vi "Renishaw-XL80_SetAutoCompensationMode.vi"(8 "error in (no error)":errorcluster, 10 "AutoCompensationMode":i32(ring) items=["AUTO_COMPENSATION_OFF"=0, "AUTO_COMPENSATION_AIR"=1, "AUTO_COMPENSATION_FULL"=3], 11 "Renishaw-XL80 in":refnum<class "Renishaw-XL80.lvclass">) -> (0 "error out":errorcluster, 3 "Renishaw-XL80 out":refnum<class "Renishaw-XL80.lvclass">)   [LabVIEW 2024, in "Renishaw-XL80.lvclass"]
doc: "Writing this property will set the current compensation mode.\n\nDefinition\nHRESULT\nput_AutoCompensationMode(\n [in] AUTO_COMPENSATION_MODES newVal\n);\nParameters\nnewVal\nSpecifies the compensation mode to use. Must be one of the values specified by the enumerated type AUTO_COMPENSATION_MODES.\n\nComments\nThis property will return with an HRESULT of E_INVALIDARG if newVal specifies a value that is not a member of the enumerated type AUTO_COMPENSATION_MODES.\n\nThis property will return with an HRESULT of E_FAIL if the current MeasurementMode is set to MEASUREMENT_ANGULAR and newVal is set to AUTO_COMPENSATION_FULL.\n\nIf the client sets AutoCompensationMode to AUTO_COMPENSATION_FULL then both lambda and the material compensation factor will be updated immediately and then automatically as new environmental values arrive.\n\nIf the client sets AutoCompensationMode to AUTO_COMPENSATION_AIR then lambda will be updated immediately and then automatically as new environmental values arrive. The material compensation factor will no longer be updated automatically. It will remain at its last updated value.\n\nIf the client sets AutoCompensationMode to AUTO_COMPENSATION_OFF then lambda and the material compensation factor will cease to be updated automatically. They will remain at their last updated values.\n\nIf the property is successful it will return with an HESULT of S_OK."
uses:
  Renishaw-XL80.lvclass
  Renishaw-XL80.lvclass/Renishaw-XL80.ctl
  D:/A.C.M/Example CSharp_64/bin/Debug/Interop.DX10SDKADAPTORLib.dll
  Example CSharp_64/bin/Debug/Interop.DX10SDKADAPTORLib.dll
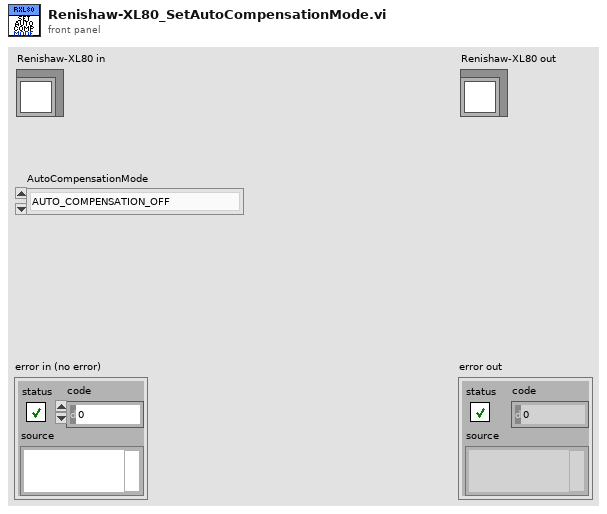
[diagram p1: front panel]
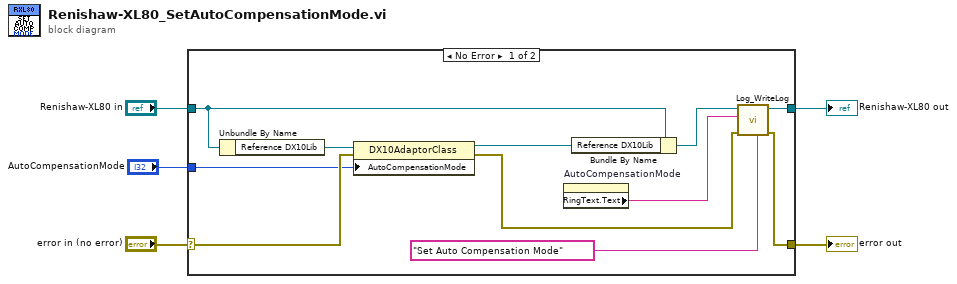
[diagram p0: block diagram]
diagram:
  n1 = case shown="No Error" "error in (no error)" {
    selector: "error in (no error)" -> [w14 w18]
    tunnel: [w8 w18] -> w4
    tunnel: [w9 w17] -> w2
    tunnel: "Renishaw-XL80 in" -> [w13 w17]
    tunnel: "AutoCompensationMode" -> [w12 _]
    frame No Error {
      n2 = Unbundle By Name(w13) -> ("Reference DX10Lib"=w16:refnum<k24>)
      n3 = property class="DX10AdaptorClass"(reference=w16, error in=w14, "AutoCompensationMode"=w12) -> (reference out=w15:refnum<k24>, error out=w6:errorcluster)
      n4 = property on="AutoCompensationMode" class="Ring (strict)"() -> ("RingText.Text"=w11:string)  [unwired: 2 in, 2 out]
      n5 = Bundle By Name(cluster=w13, "Reference DX10Lib"=w15) -> (w10:refnum<class "Renishaw-XL80.lvclass">)
      n6 = call-dynamic "Log_WriteLog.vi"("Additional text"="Set Auto Compensation Mode", "error in (no error)"=w6, "Command"=w11, "Log in"=w10) -> ("error out"=w8:errorcluster, "Log out"=w9:refnum<class "Renishaw-XL80.lvclass">)  [unwired: 6 in]
    }
    frame Error {
    }
  }
  "error out" <- w4
  "Renishaw-XL80 out" <- w2
